vi "polar.vi"() -> ()   [LabVIEW 2016]
panel:
  in  "magnitude":dbl[](array[numeric])=[3.0, 3.2, 3.4, 3.6, 4.2, 5.0, 5.3, 5.4, 5.3, 4.8, 4.2, 4.1, 4.3, 4.9, 5.3, 5.4, 5.3, 4.9, 4.6, 4.2, 3.6, 3.0, 2.4, 2.0, 1.5, 1.0, 0.9, 0.7, 0.4, 0.1, 0.05, 0.0, 0.1, 0.2, 0.4, 0.6, 0.8, 1.0]
  in  "angle":dbl[](array[numeric])=[0.0, 0.0, 10.0, 20.0, 30.0, 40.0, 50.0, 60.0, 70.0, 80.0, 90.0, 100.0, 110.0, 120.0, 130.0, 140.0, 150.0, 160.0, 170.0, 180.0, 190.0, 200.0, 210.0, 220.0, 230.0, 240.0, 250.0, 260.0, 270.0, 280.0, 290.0, 300.0, 310.0, 320.0, 330.0, 340.0, 350.0, 360.0]
  in  "polar attributes":T1={"maximum"=0.0, "minimum"=0.0, "clip to min"=FALSE, "log?(F)"=FALSE, "grid color"=6710886, "plot color"=16711680, "fmt and prec"={"format"=enum."Decimal", "precision"=0}, "visible section"=8} {"minimum" format="%0.2f"; "maximum" format="%0.2f"}
  out "XY Graph":cluster{dbl[], dbl[]}(graph)={[0.0, 0.0, 10.0, 20.0, 30.0, 40.0, 50.0, 60.0, 70.0, 80.0, 90.0, 100.0, 110.0, 120.0, 130.0, 140.0, 150.0, 160.0, 170.0, 180.0, 190.0, 200.0, 210.0, 220.0, 230.0, 240.0, 250.0, 260.0, 270.0, 280.0, 290.0, 300.0, 310.0, 320.0, 330.0, 340.0, 350.0, 360.0], [3.0, 3.2, 3.4, 3.6, 4.2, 5.0, 5.3, 5.4, 5.3, 4.8, 4.2, 4.1, 4.3, 4.9, 5.3, 5.4, 5.3, 4.9, 4.6, 4.2, 3.6, 3.0, 2.4, 2.0, 1.5, 1.0, 0.9, 0.7, 0.4, 0.1, 0.05, 0.0, 0.1, 0.2, 0.4, 0.6, 0.8, 1.0]}
  out "Polar Plot":picture
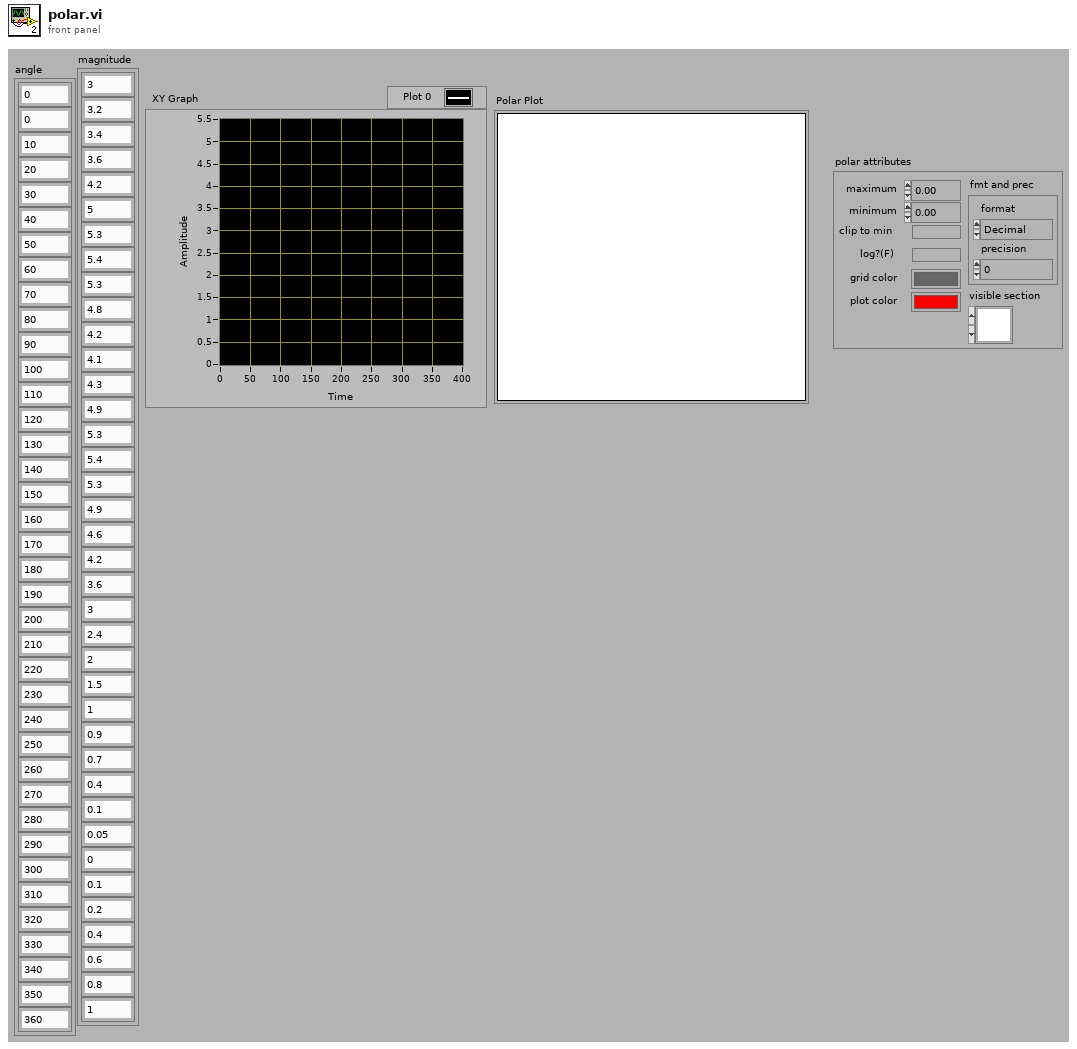
[diagram p1: front panel]
types:
  T1 = cluster{"maximum":dbl, "minimum":dbl, "clip to min":bool, "log?(F)":bool, "grid color":u32, "plot color":u32, "fmt and prec":cluster{"format":enum8{"Decimal", "Scientific", "Engineering", "Binary", "Octal", "Hex"}, "precision":u8}, "visible section":u16}
  T2 = typedef "LVBoundsTypeDef.ctl" = cluster{"Width":u32, "Height":u32}
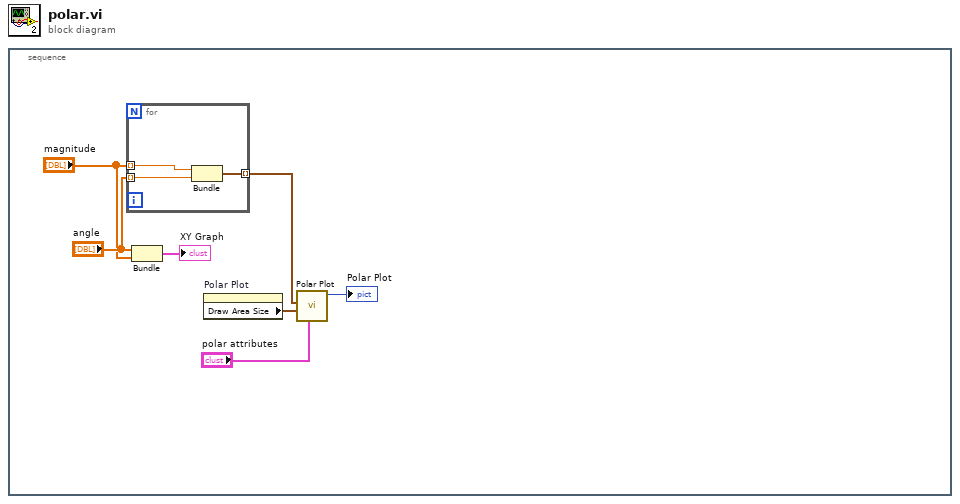
[diagram p0: block diagram]
diagram:
  n1 = stacked-sequence {
    frame #0 {
      n2 = for {
        tunnel: "magnitude" -> [w10] mode=indexing
        tunnel: "angle" -> [w9] mode=indexing
        tunnel: [w8] -> w5 mode=indexing
        n3 = Bundle("magnitude"=w10, "phase"=w9) -> (w8:cluster{"magnitude":dbl, "phase":dbl})  [unwired: 1 in]
      }
      n4 = Bundle("angle"="angle", "magnitude"="magnitude") -> (→"XY Graph":cluster{"angle":dbl[], "magnitude":dbl[]})  [unwired: 1 in]
      n5 = property on="Polar Plot" class="Pict"() -> ("Draw Area Size"=w2:T2)  [unwired: 2 in, 2 out]
      n6 = call <vilib>:"Polar Plot.vi"("polar attributes"="polar attributes", "dimensions (w,h)"=w2, "data array [mag, phase (deg)]"=w5) -> ("new picture"=→"Polar Plot":picture)  [unwired: 8 in]
    }
  }
